vi "Transfer File.vi"(8 "error in (no error)":errorcluster, 9 "Dest Filename":path, 10 "Source Filename":string, 11 "VISA resource name":refnum<visa-resource-name>) -> (0 "error out":errorcluster, 3 "VISA resource name out":refnum<visa-resource-name>)   [LabVIEW 2013, in "LeCroy Wave Series.lvlib"]
doc: "Transfers a file from the oscilloscope's hard drive to a destination filepath on the remote PC. If the destination filename already exists, then the file isn't saved."
uses:
  LeCroy Wave Series.lvlib
panel:
  out "File data":string
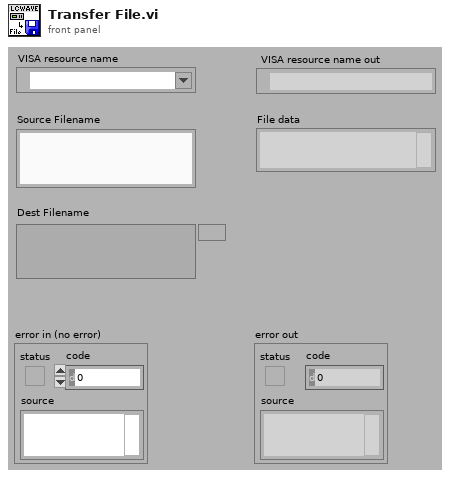
[diagram p1: front panel]
types:
  T1 = enum16{"open", "open or create", "create or replace", "create", "open (read only)"}
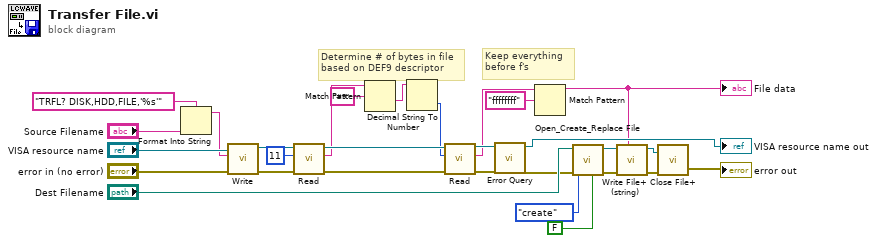
[diagram p0: block diagram]
diagram:
  # "Keep everything \nbefore f's"
  # "Determine # of bytes in file\nbased on DEF9 descriptor"
  n1 = Format Into String(format string="TRFL? DISK,HDD,FILE,'%s'" ("initial string"), "Source Filename") -> (resulting string=w25:string)  [unwired: 2 in, 1 out]
  n2 = call "Write.vi"("error in (no error)"="error in (no error)", "Write Buffer"=w25, "VISA resource name"="VISA resource name") -> ("error out"=w21:errorcluster, "VISA resource name out"=w24:refnum<visa-resource-name>)  [unwired: 6 in, 1 out]
  n3 = call "Read.vi"("error in (no error)"=w21, "Byte Count"=u32 11, "VISA resource name"=w24) -> ("error out"=w20:errorcluster, "Read Buffer"=w18:string, "VISA resource name out"=w23:refnum<visa-resource-name>)  [unwired: 5 in, 1 out]
  n4 = Match Pattern(string=w18, regular expression="#9") -> (after substring=w16:string)  [unwired: 1 in, 3 out]
  n5 = Decimal String To Number(string=w16) -> (number=w15:i32)  [unwired: 2 in, 1 out]
  n6 = call "Read.vi"("error in (no error)"=w20, "Byte Count"=w15, "VISA resource name"=w23) -> ("error out"=w7:errorcluster, "Read Buffer"=w13:string, "VISA resource name out"=w22:refnum<visa-resource-name>)  [unwired: 5 in, 1 out]
  n7 = call "Error Query.vi"("error in (no error)"=w7, "VISA resource name"=w22) -> ("error out"=w6:errorcluster, "VISA resource name out"=→"VISA resource name out":refnum<visa-resource-name>)  [unwired: 6 in, 2 out]
  n8 = Match Pattern(string=w13, regular expression="ffffffff") -> (before substring=w1:string)  [unwired: 1 in, 3 out]
  "File data" <- w1
  n9 = call <vilib>:"Open_Create_Replace File.vi"("advisory dialog? (display:T)"=FALSE, "error in (no error)"=w6, "function (open:0)"=T1."create", "file path"="Dest Filename") -> ("error out"=w11:errorcluster, "refnum"=w5:refnum<file>)  [unwired: 4 in, 2 out]
  n10 = call <vilib>:"Write File+ (string).vi"("string"=w1, "error in (no error)"=w11, "refnum"=w5) -> ("error out"=w10:errorcluster, "dup refnum"=w4:refnum<file>)  [unwired: 4 in, 1 out]
  n11 = call <vilib>:"Close File+.vi"("error in (no error)"=w10, "refnum"=w4) -> ("error out"=→"error out":errorcluster)  [unwired: 3 in, 2 out]
